vi "Update Parameter VS Channels.vi"(8 "error in (no error)":errorcluster, 10 "From HWIn Buf":dbl[](array[numeric]), 11 "Label Settings":T1 {"Words"."Param Setting"."Num Bits" min=1 max=32; "Words"."Param Setting"."Start Bit" min=8 max=31; "Words"."Block Data Refs"."Data Reference" format="%.0x"; "Label" format="%.0o"}) -> (0 "error out":errorcluster, 3 "Label Settings":T1 {"Words"."Param Setting"."Num Bits" min=1 max=32; "Words"."Param Setting"."Start Bit" min=8 max=31; "Words"."Block Data Refs"."Data Reference" format="%.0x"; "Label" format="%.0o"})   [LabVIEW 2011, in "AIT 429 Custom Device.lvlib"]
uses:
  AIT 429 Custom Device.lvlib
  RT Controls/RT Label Settings.ctl
  Controls and Global/Label.ctl
  Controls and Global/transferPeriod.ctl
  RT Controls/Driver Data.ctl
  RT Controls/RT Word Settings.ctl
  <vilib>/NI Veristand/Custom Device API/Block Data Reference.ctl
  <vilib>/NI Veristand/Custom Device API/Data Reference.ctl
  RT Controls/RT Param Setting.ctl
  Controls and Global/Start Bit.ctl
  Controls and Global/Number of Bits.ctl
  Controls and Global/TransferType.ctl
  <vilib>/NI Veristand/Custom Device API/Global Data Refs.vi
  <vilib>/NI Veristand/Custom Device API/Custom Device API.lvlib
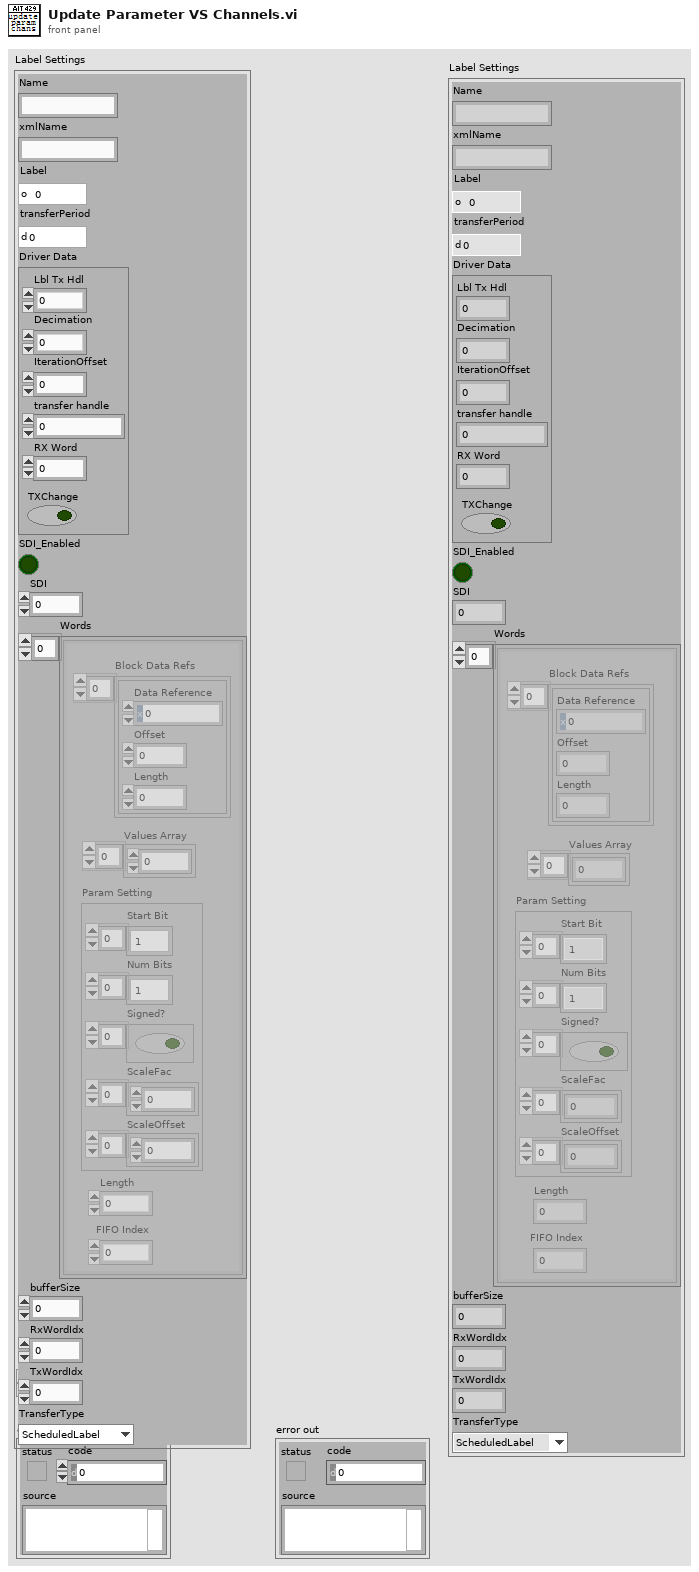
[diagram p1: front panel]
types:
  T1 = typedef "AIT 429 Custom Device.lvlib/RT Label Settings.ctl" = cluster{"Name":string, "xmlName":string, "Label":T2, "transferPeriod":T3, "Driver Data":T4, "SDI_Enabled":bool, "SDI":u8, "Words":T5[], "bufferSize":u32, "RxWordIdx":i32, "TxWordIdx":i32, "TransferType":T11}
  T2 = typedef "AIT 429 Custom Device.lvlib/Label.ctl" = u8
  T3 = typedef "AIT 429 Custom Device.lvlib/transferPeriod.ctl" = u32
  T4 = typedef "AIT 429 Custom Device.lvlib/Driver Data.ctl" = cluster{"Lbl Tx Hdl":u32, "Decimation":i32, "IterationOffset":i32, "transfer handle":u32, "RX Word":u32, "TXChange":bool}
  T5 = typedef "AIT 429 Custom Device.lvlib/RT Word Settings.ctl" = cluster{"Block Data Refs":T6[], "Values Array":dbl[], "Length":i32, "FIFO Index":i32, "Param Setting":T8}
  T6 = typedef "Custom Device API.lvlib/Block Data Reference.ctl" = cluster{"Data Reference":T7, "Offset":i32, "Length":i32}
  T7 = typedef "Custom Device API.lvlib/Data Reference.ctl" = i32
  T8 = typedef "AIT 429 Custom Device.lvlib/Rt Param Setting.ctl" = cluster{"Start Bit":T9[], "Num Bits":T10[], "Signed?":bool[], "ScaleFac":dbl[], "ScaleOffset":dbl[]}
  T9 = typedef "AIT 429 Custom Device.lvlib/Start Bit.ctl" = i32
  T10 = typedef "AIT 429 Custom Device.lvlib/Number of Bits.ctl" = i32
  T11 = typedef "AIT 429 Custom Device.lvlib/TransferType.ctl" = enum16{"ScheduledLabel", "Acyclic", "Block", "Strobe"}
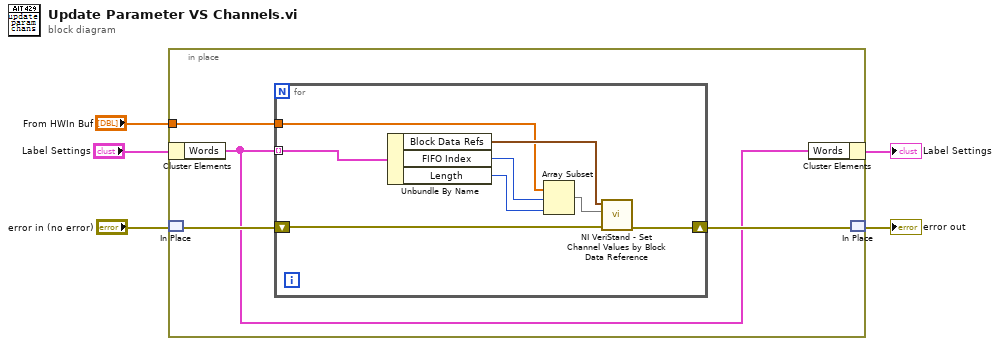
[diagram p0: block diagram]
diagram:
  n1 = in-place {
    in-place-border: "From HWIn Buf" -> [w9]
    n2 = in-place-cluster #1("Label Settings") -> ("Words"=w6:T5[])
    n3 = in-place-match #2("error in (no error)") -> (w8:errorcluster)
    n4 = for {
      tunnel: w9 -> [w14]
      tunnel: w6 -> [w13] mode=indexing
      shift-right: [w11] -> w7
      shift-left: w8 -> [w12]
      n5 = Unbundle By Name(w13) -> ("Block Data Refs"=w16:T6[], "FIFO Index"=w15:i32, "Length"=w10:i32)
      n6 = Array Subset(array=w14, index=w15, length=w10) -> (w17:dbl[])
      n7 = call <vilib>:"NI VeriStand - Set Channel Values by Block Data Reference.vi"("error in (no error)"=w12, "Values Array in"=w17, "Block Data Ref"=w16) -> ("error out"=w11:errorcluster)  [unwired: 6 in, 2 out]
    }
    n8 = in-place-cluster #1("Words"=w6) -> (→"Label Settings":T1)
    n9 = in-place-match #2(w7) -> (→"error out":errorcluster)
  }
